vi "SplashWnd - Module Starting Up3.vi"(5 "Background VI Ref (Callee's Caller)":refnum<vi>, 6 "LoadingWait(ms)":u32=100, 7 "Title":string, 8 "Error In (No Error)":errorcluster, 9 "Name (\"\" to Use UUID)":string="SplashWindow") -> (0 "error out":errorcluster)   [LabVIEW 2020]
uses:
  csm/CSM-Utils/CSM-ModuleManager/Operation.ctl
  79d02799-5e27-450a-8f22-22593f2d7556.vi
  csm/CSM-ModSets-SplashWindow/SplashWindow.vi
  <userlib>/_NEVSTOP/Communicable State Machine(CSM)/addons/API-String-Arugments-Support/_Support/Data To API String Arguments.vi
  csm/CSM-ModSets-SplashWindow/CSM-SplashWindow.lvlib
  <userlib>/_NEVSTOP/Communicable State Machine(CSM)/Communicable State Machine.lvlib
  <userlib>/_NEVSTOP/Communicable State Machine(CSM)/addons/INI-Static-Variable-Support/INI-Static-Variable-Support.lvlib
  csm/CSM-Utils/CSM-ModuleManager/CSM-ModuleManager.lvlib
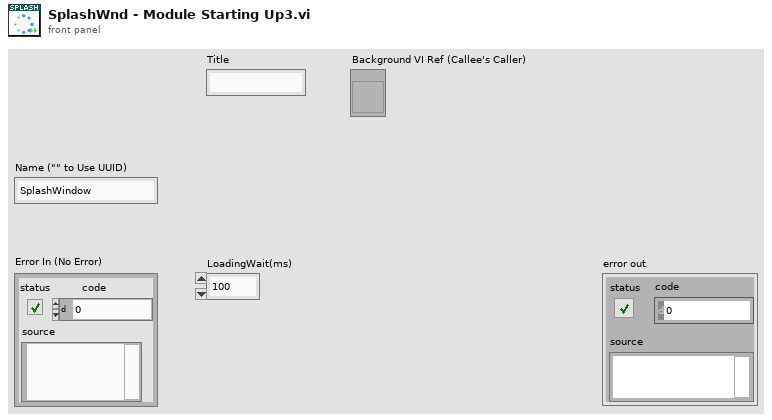
[diagram p1: front panel]
types:
  T1 = typedef "CSM-ModuleManager.lvlib/Operation.ctl" = enum16{"Register", "UnRegister", "Load Config", "Get"}
  T2 = enum32{"Invalid", "Default", "Floating", "Floating/Auto-Hide", "Modal"}
  T3 = enum32{"Invalid", "Standard", "Closed", "Hidden", "Minimized", "Maximized"}
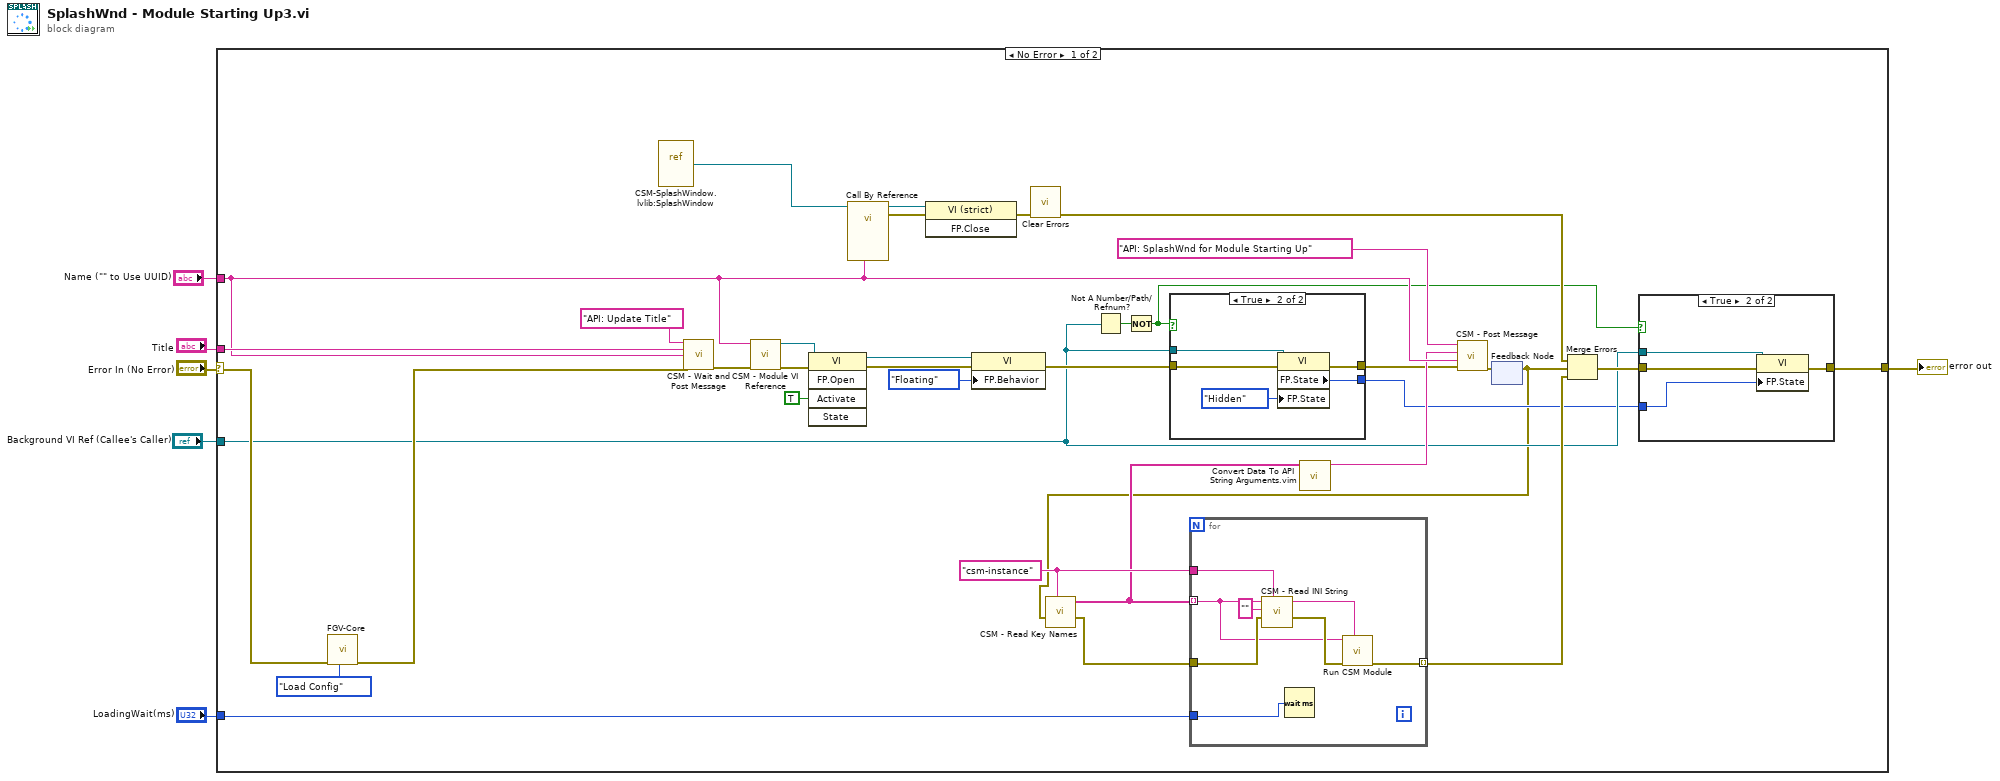
[diagram p0: block diagram]
diagram:
  n1 = case shown="No Error" "Error In (No Error)" {
    selector: "Error In (No Error)" -> [w22 w61]
    tunnel: "Title" -> [w41 _]
    tunnel: [w14 w61] -> w4
    tunnel: "Name (\"\" to Use UUID)" -> [w40 _]
    tunnel: "Background VI Ref (Callee's Caller)" -> [w12 _]
    tunnel: "LoadingWait(ms)" -> [w10 _]
    frame No Error {
      w23 = "csm-instance" ("Section Name (\"\" as Default)")
      n2 = call "FGV-Core.vi"("Enum"=Operation."Load Config", "error in (no error)"=w22) -> ("error out"=w19:errorcluster)  [unwired: 7 in, 2 out]
      n3 = vi-ref "CSM-SplashWindow.lvlib:SplashWindow.vi"() -> (w18:refnum<vi>)
      n4 = call <userlib>:"CSM - Wait and Post Message.vi"("State"="API: Update Title", "Arguments (\"\")"=w41, "Target Module"=w40, "Error In (No Error)"=w19) -> ("error out"=w38:errorcluster)  [unwired: 10 in, 1 out]
      n5 = call <userlib>:"CSM - Module VI Reference.vi"("error in (no error)"=w38, "CSM Name"=w40) -> ("error out"=w36:errorcluster, "CSM Module VIRef"=w37:refnum<vi>)  [unwired: 8 in]
      n6 = invoke class="VI" method="FP.Open"(reference=w37, error in=w36, "Activate"=TRUE ("Activate?")) -> (reference out=w34:refnum<vi>, error out=w35:errorcluster)  [unwired: 2 in, 3 out]
      n7 = call-by-ref "?"(reference=w18, "Name (\"\" to Use UUID)"=w40) -> (reference out=w27:refnum<vi>, error out=w31:errorcluster)  [unwired: 12 in]
      n8 = invoke class="VI (strict)" method="FP.Close"(reference=w27, error in=w31) -> (error out=w28:errorcluster)  [unwired: 1 in, 2 out]
      n9 = property class="VI"(reference=w34, error in=w35, "FP.Behavior"=T2."Floating" ("Front Panel Window:Behavior")) -> (error out=w16:errorcluster)  [unwired: 1 out]
      n10 = call <vilib>:"Clear Errors.vi"("error in (no error)"=w28) -> ("error out"=w26:errorcluster)  [unwired: 5 in, 1 out]
      n11 = Not A Number/Path/Refnum?(number/path/refnum=w12) -> (NaN/Path/Refnum?=w17:bool)
      n12 = Not(x=w17) -> (.not. x?=w13:bool)
      n13 = case shown="True" w13 {
        tunnel: w16 -> [w47 w52]
        tunnel: [w47 w50] -> w9
        tunnel: w12 -> [_ w51]
        tunnel: [_ w48] -> w11
        frame False {
        }
        frame True {
          n14 = property class="VI"(reference=w51, error in=w52, "FP.State"=T3."Hidden" ("Front Panel Window:State")) -> (error out=w50:errorcluster, "FP.State"=w48:T3)  [unwired: 1 out]
        }
      }
      n15 = feedback #1() -> (w7:errorcluster)  [unwired: 1 in]
      n16 = call <userlib>:"CSM - Read Key Names.vi"("Section Name (\"\" as Default)"=w23, "error in (no error)"=w7) -> ("error out"=w25:errorcluster, "Keys"=w21:string[])  [unwired: 6 in]
      n17 = for {
        tunnel: w23 -> [w59]
        tunnel: w21 -> [w54] mode=indexing
        tunnel: w25 -> [w60]
        tunnel: [w56] -> w20 mode=indexing
        tunnel: w10 -> [w53]
        n18 = call <userlib>:"CSM - Read INI String.vi"("Section Name (\"\" as Default)"=w59, "error in (no error)"=w60, "Default Value"="", "Variable Name"=w54) -> ("error out"=w57:errorcluster, "Value"=w55:string)  [unwired: 3 in, 1 out]
        n19 = Wait (ms)(milliseconds to wait=w53) -> ()  [unwired: 1 out]
        n20 = call "Run CSM Module.vi"("CSM-Module"=w55, "Error in"=w57, "CSM-Instance"=w54) -> ("Error out"=w56:errorcluster)  [unwired: 8 in]
      }
      n21 = call "Convert Data To API String Arguments.vim"("Data"=w21) -> ("API String"=w30:string)  [unwired: 7 in, 1 out]
      n22 = call <userlib>:"CSM - Post Message.vi"("Error In (No Error)"=w9, "Target Module"=w40, "Arguments (\"\")"=w30, "State"="API: SplashWnd for Module Starting Up") -> ("error out"=w8:errorcluster)  [unwired: 7 in]
      n23 = feedback-in #1(w8) -> ()
      n24 = Merge Errors(w26, w7, w20) -> (w15:errorcluster)
      n25 = case shown="True" w13 {
        tunnel: w15 -> [w42 w46]
        tunnel: [w42 w44] -> w14
        tunnel: w12 -> [_ w45]
        tunnel: w11 -> [_ w43]
        frame False {
        }
        frame True {
          n26 = property class="VI"(reference=w45, error in=w46, "FP.State"=w43) -> (error out=w44:errorcluster)  [unwired: 1 out]
        }
      }
    }
    frame Error {
    }
  }
  "error out" <- w4
